vi "1.5 Log.vi"(8 "error in (no error)":errorcluster caption="错误输入（无错误）", 10 "Log Msg":string="test log", 11 "路径":path=path "D:/") -> (0 "错误输出":errorcluster)   [LabVIEW 2018]
doc: "Log:xxx\n1.\n2."
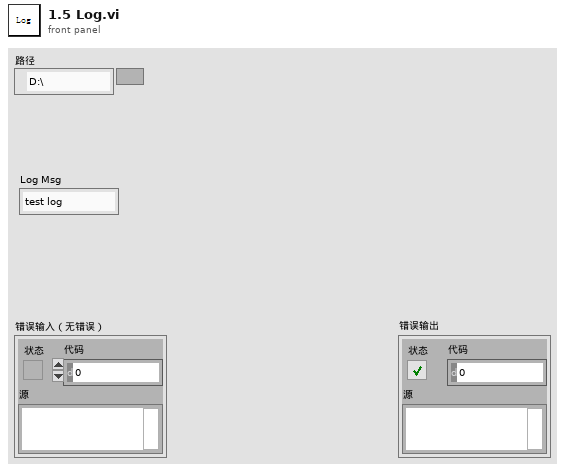
[diagram p1: front panel]
types:
  T1 = enum16{"open", "replace", "create", "open or create", "replace or create", "replace or create with confirmation"}
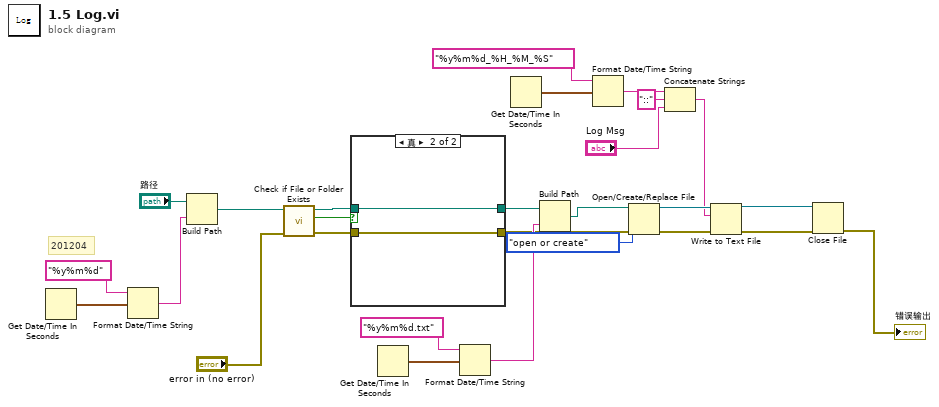
[diagram p0: block diagram]
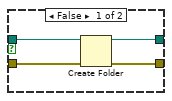
[diagram p2: hidden frame]
diagram:
  # "201204"
  n1 = Get Date/Time In Seconds() -> (seconds since 1Jan1904=w26:timestamp)
  n2 = Format Date/Time String(time format string (%c)="%y%m%d" ("时间格式字符串(%c)"), seconds (now)=w26) -> (date/time string=w24:string)  [unwired: 1 in]
  n3 = Build Path(base path="路径", name or relative path=w24) -> (appended path=w23:path)
  n4 = call <vilib>:"Check if File or Folder Exists.vi"("error in (no error)"="error in (no error)", "path"=w23) -> ("error out"=w20:errorcluster, "file or folder exists?"=w22:bool, "dup path"=w21:path)  [unwired: 7 in]
  n5 = case shown="真" w22 {
    tunnel: w21 -> [w31 w33]
    tunnel: w20 -> [w30 w32]
    tunnel: [w29 w33] -> w19
    tunnel: [w28 w32] -> w14
    frame False {
      n6 = Create Folder(path (use dialog)=w31, error in=w30) -> (created path=w29:path, error out=w28:errorcluster)  [unwired: 1 in, 1 out]
    }
    frame True {
    }
  }
  n7 = Get Date/Time In Seconds() -> (seconds since 1Jan1904=w17:timestamp)
  n8 = Format Date/Time String(time format string (%c)="%y%m%d.txt" ("时间格式字符串(%c)"), seconds (now)=w17) -> (date/time string=w16:string)  [unwired: 1 in]
  n9 = Get Date/Time In Seconds() -> (seconds since 1Jan1904=w8:timestamp)
  n10 = Build Path(base path=w19, name or relative path=w16) -> (appended path=w15:path)
  n11 = Format Date/Time String(time format string (%c)="%y%m%d_%H_%M_%S" ("时间格式字符串(%c)"), seconds (now)=w8) -> (date/time string=w6:string)  [unwired: 1 in]
  n12 = Open/Create/Replace File(file path (use dialog)=w15, error in=w14, operation (0:open)=T1."open or create" ("操作(0:open)")) -> (refnum out=w12:refnum<file>, error out=w11:errorcluster)  [unwired: 3 in, 1 out]
  n13 = Concatenate Strings(w6, "::" ("字符串"), "Log Msg") -> (w3:string)
  n14 = Write to Text File(file (use dialog)=w12, text=w3, error in=w11) -> (refnum out=w10:refnum<file>, error out=w9:errorcluster)  [unwired: 1 in, 1 out]
  n15 = Close File(refnum=w10, error in=w9) -> (error out=→"错误输出":errorcluster)  [unwired: 1 out]
